vi "Write_raw_block_header.vi"(0 "No of LDA samples":i32, 1 "No of analogue samples":i32, 2 "Block Timings":T1={"Started"=0.0, "Ended"=0.0, "Analogue Frequency Hz"=1000.0} {"Analogue Frequency Hz" format="%.2f"}, 3 "No of PWA samples":i32, 4 "Add to Block Header":string) -> (5 "Output string":string)   [LabVIEW 2010]
uses:
  Controls/Block_start_and_end.ctl
  Globals/Meas_global.vi
  Globals/LDA_meas_global_1.vi
  Globals/Plug_in_data_global.vi
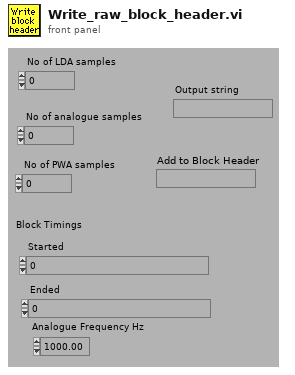
[diagram p1: front panel]
types:
  T1 = typedef "Block_start_and_end.ctl" = cluster{"Started":dbl, "Ended":dbl, "Analogue Frequency Hz":dbl}
  T2 = cluster{"scale multiplier":dbl, "scale offset":dbl}[]
  T3 = typedef "Ch_description_ADAM.ctl" = cluster{"Ch Name":string, "Type":T4, "Function":T5, "Ch State":T6, "Calibration type":T7, "A":dbl, "B":dbl, "C":dbl, "D":dbl, "Comments":string, "Address":T8, "String":string, "Duty":u16}
  T4 = typedef "Module_type_ADAM.ctl" = enum16{"4011", "4012", "4013", "4014", "4016", "4017", "4018", "4021", "4050", "4052", "4053", "4060", "4080", "5000", "5017", "5018", "5024", "5051", "5056", "5060", "6060", "Tracker", "WEST", "GILL", "JEM", "VICI", "Vaisala", "DRUCK", "Run VI Named:", "IR2100", "PPT", "Comparator", "VIRTUAL", "Hold Value", "Read A", "Read Ch", "Coded", "Client Info", "Web Client", "X10", "Test"}
  T5 = typedef "Function_ADAM.ctl" = enum16{"Analogue Input", "Digital Input", "Event counter", "Event rate", "Analogue Output", "Digital Output", "Relay Output"}
  T6 = typedef "Channel_State.ctl" = enum16{"On", "Off", "Always On", "Always Off"}
  T7 = typedef "Calib_type_ADAM.ctl" = enum16{"Raw", "Bx + A", "Cx^2 + Bx + A", "Dx^3 + Cx^2 + Bx + A", "In Band", "Hi-Tec Q", "Hi-Tec M_dot", "Text"}
  T8 = typedef "Address.ctl" = cluster{"Main":i32, "Ch.":i32, "Sub":i32, "Port Name":string}
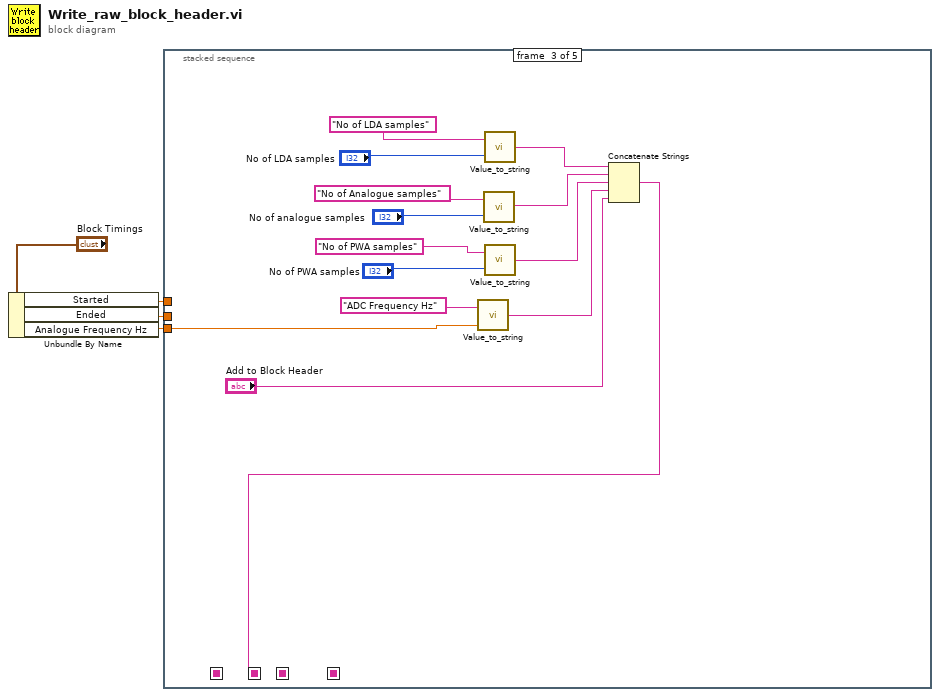
[diagram p0: block diagram]
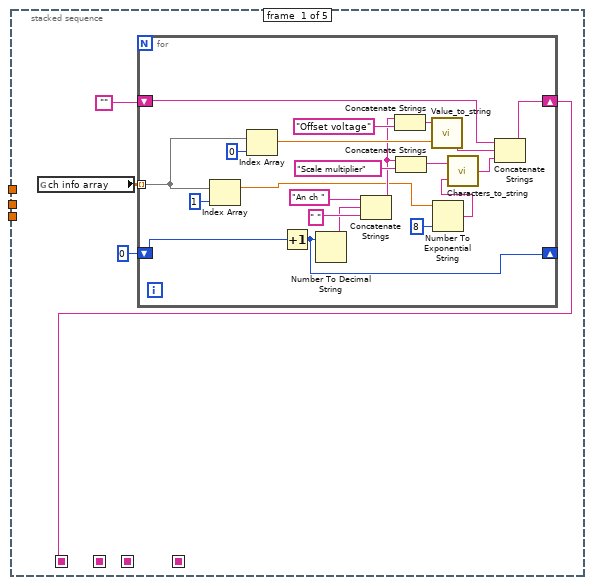
[diagram p2: hidden frame]
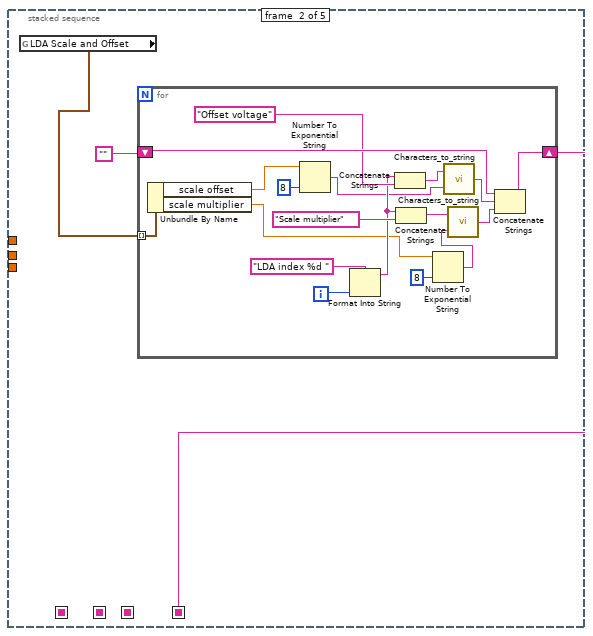
[diagram p3: hidden frame]
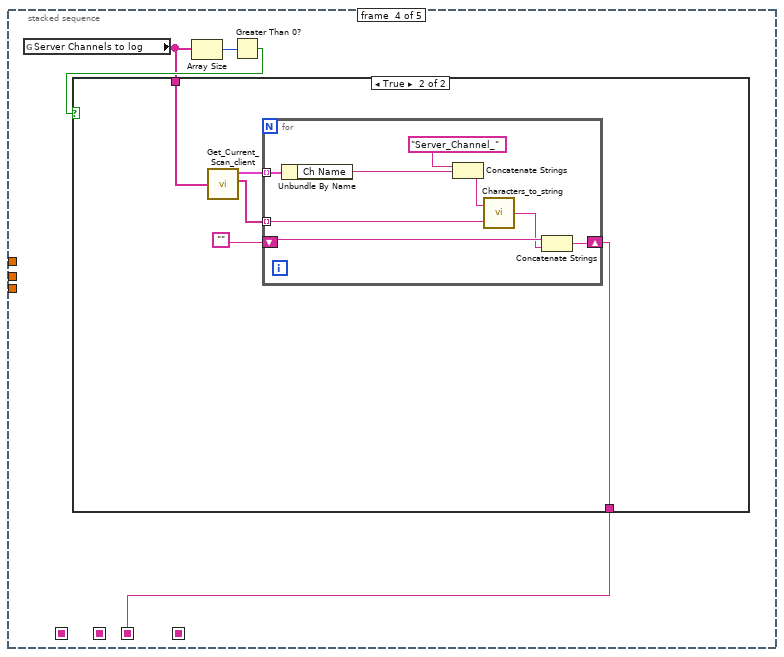
[diagram p4: hidden frame]
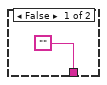
[diagram p5: hidden frame]
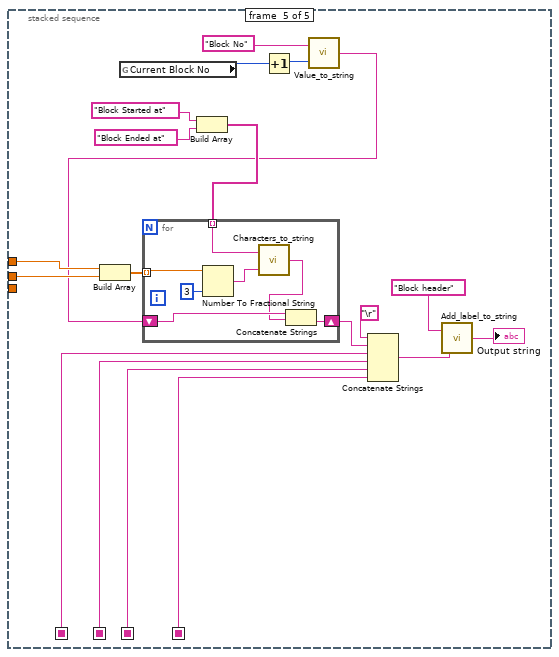
[diagram p6: hidden frame]
diagram:
  n1 = Unbundle By Name("Block Timings") -> ("Started"=w3:dbl, "Ended"=w2:dbl, "Analogue Frequency Hz"=w1:dbl)
  n2 = stacked-sequence {
    seq-local: [w5 _ _ _ _] -> [_ _ _ _ w100]
    seq-local: [_ _ w58 _ _] -> [_ _ _ _ w99]
    seq-local: [_ _ _ w65 _] -> [_ _ _ _ w84]
    seq-local: [_ w30 _ _ _] -> [_ _ _ _ w83]
    tunnel: w3 -> [_ _ _ _ w92]
    tunnel: w2 -> [_ _ _ _ w91]
    tunnel: w1 -> [_ _ w57 _ _]
    frame #0 {
      n3 = global read "Meas_global.vi" "ch info array"() -> (w7:dbl[][])
      n4 = for {
        shift-right: [w28] -> w5
        shift-left: "" -> [w29]
        tunnel: w7 -> [w27] mode=indexing
        shift-right: [w25] -> _
        shift-left: 0 -> [w26]
        n5 = Index Array(array=w27, index=1) -> (element=w9:dbl)
        n6 = Index Array(array=w27, index=0) -> (element=w18:dbl)
        n7 = Increment(x=w26) -> (x+1=w25:i32)
        n8 = Number To Decimal String(number=w25) -> (decimal integer string=w15:string)  [unwired: 1 out]
        n9 = Concatenate Strings("An ch ", w15, " ") -> (w14:string)
        n10 = Concatenate Strings(w14, "Offset voltage") -> (w22:string)
        n11 = Concatenate Strings(w14, "Scale multiplier") -> (w11:string)
        n12 = call "Value_to_string.vi"("Value"=w18, "Label for value"=w22) -> ("Output string"=w24:string)  [unwired: 1 in]
        n13 = Number To Exponential String(number=w9, precision (6)=i16 8) -> (E-format string=w10:string)  [unwired: 2 out]
        n14 = call "Characters_to_string.vi"("Characters to write"=w10, "Label for characters"=w11) -> ("Output string"=w12:string)
        n15 = Concatenate Strings(w29, w24, w12) -> (w28:string)
      }
    }
    frame #1 {
      n16 = global read "LDA_meas_global_1.vi" "LDA Scale and Offset"() -> (w31:T2)
      n17 = for {
        shift-right: [w49] -> w30
        shift-left: "" -> [w50]
        tunnel: w31 -> [w42] mode=indexing
        i -> [w39]
        n18 = Unbundle By Name(w42) -> ("scale offset"=w35:dbl, "scale multiplier"=w38:dbl)
        n19 = Number To Exponential String(number=w35, precision (6)=i16 8) -> (E-format string=w34:string)  [unwired: 2 out]
        n20 = Format Into String(format string="LDA index %d ", w39) -> (resulting string=w40:string)  [unwired: 2 in, 1 out]
        n21 = Concatenate Strings(w40, "Offset voltage") -> (w37:string)
        n22 = Concatenate Strings(w40, "Scale multiplier") -> (w44:string)
        n23 = Number To Exponential String(number=w38, precision (6)=i16 8) -> (E-format string=w43:string)  [unwired: 2 out]
        n24 = call "Characters_to_string.vi"("Characters to write"=w34, "Label for characters"=w37) -> ("Output string"=w33:string)
        n25 = call "Characters_to_string.vi"("Characters to write"=w43, "Label for characters"=w44) -> ("Output string"=w45:string)
        n26 = Concatenate Strings(w50, w33, w45) -> (w49:string)
      }
    }
    frame #2 {
      n27 = call "Value_to_string.vi"("Value"=w57, "Label for value"="ADC Frequency Hz") -> ("Output string"=w52:string)  [unwired: 1 in]
      n28 = call "Value_to_string.vi"("Value"="No of analogue samples", "Label for value"="No of Analogue samples") -> ("Output string"=w59:string)  [unwired: 1 in]
      n29 = call "Value_to_string.vi"("Value"="No of LDA samples", "Label for value"="No of LDA samples") -> ("Output string"=w60:string)  [unwired: 1 in]
      n30 = call "Value_to_string.vi"("Value"="No of PWA samples", "Label for value"="No of PWA samples") -> ("Output string"=w53:string)  [unwired: 1 in]
      n31 = Concatenate Strings(w60, w59, w53, w52, "Add to Block Header") -> (w58:string)
    }
    frame #3 {
      n32 = global read "Plug_in_data_global.vi" "Server Channels to log"() -> (w66:string[])
      n33 = Array Size(array=w66) -> (size(s)=w68:i32)
      n34 = Greater Than 0?(x=w68) -> (x > 0?=w67:bool)
      n35 = case shown="True" w67 {
        tunnel: w66 -> [_ w73]
        tunnel: ["" w70] -> w65
        frame False {
        }
        frame True {
          n36 = call "Get_Current_Scan_client.vi"("ADAM Ch Names"=w73) -> ("Ch Description Array"=w72:T3[], "String values"=w71:string[])  [unwired: 2 out]
          n37 = for {
            shift-right: [w81] -> w70
            shift-left: "" -> [w80]
            tunnel: w72 -> [w77] mode=indexing
            tunnel: w71 -> [w75] mode=indexing
            n38 = Unbundle By Name(w77) -> ("Ch Name"=w76:string)
            n39 = Concatenate Strings("Server_Channel_" ("string"), w76) -> (w78:string)
            n40 = call "Characters_to_string.vi"("Characters to write"=w75, "Label for characters"=w78) -> ("Output string"=w79:string)
            n41 = Concatenate Strings(w80, w79) -> (w81:string)
          }
        }
      }
    }
    frame #4 {
      n42 = Build Array(w92, w91) -> (w93:dbl[])
      n43 = global read "Meas_global.vi" "Current Block No"() -> (w89:i32)
      n44 = Build Array("Block Started at", "Block Ended at") -> (w95:string[])
      n45 = Increment(x=w89) -> (x+1=w85:i32)
      n46 = call "Value_to_string.vi"("Value"=w85, "Label for value"="Block No") -> ("Output string"=w88:string)  [unwired: 1 in]
      n47 = for {
        tunnel: w95 -> [w108] mode=indexing
        shift-right: [w105] -> w97
        shift-left: w88 -> [w107]
        tunnel: w93 -> [w103] mode=indexing
        n48 = Number To Fractional String(number=w103, precision (6)=i16 3) -> (F-format string=w102:string)  [unwired: 2 out]
        n49 = call "Characters_to_string.vi"("Characters to write"=w102, "Label for characters"=w108) -> ("Output string"=w106:string)
        n50 = Concatenate Strings(w107, w106) -> (w105:string)
      }
      n51 = Concatenate Strings("\r", w97, w100, w99, w84, w83) -> (w98:string)
      n52 = call "Add_label_to_string.vi"("String to write"=w98, "File Label"="Block header") -> ("Output string"=→"Output string":string)
    }
  }
